vi "TMY_R2_set_angle.vi"() -> ()   [LabVIEW 2023, in "TMY_R2_20250714.lvlib"]
uses:
  TMY_R2_20250714.lvlib
panel:
  out "String":string
  in  "Phi":i32 min=0 max=360
  in  "Theta":i32 min=0 max=360
  in  "COM_No.":string="10"
  out "floder?":bool
  out "standard output":string
  out "standard error":string
  in  "error in":errorcluster
  in  "Func.":enum16{"Theta", "Phi"}(ring)
  out "error out":errorcluster
  # "# 設定角度\ntheta_angle = 10 #大轉盤\nphi_angle = 20 #DUT轉盤"
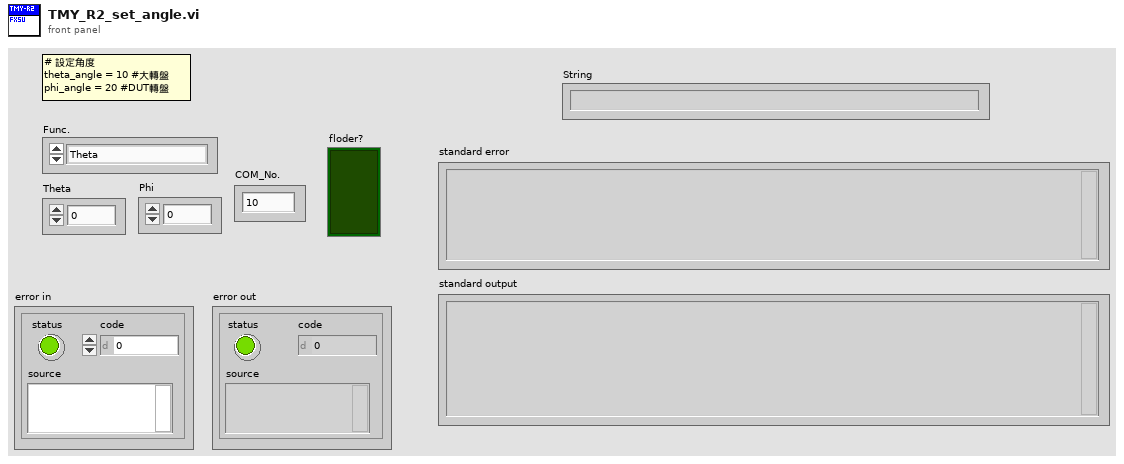
[diagram p1: front panel]
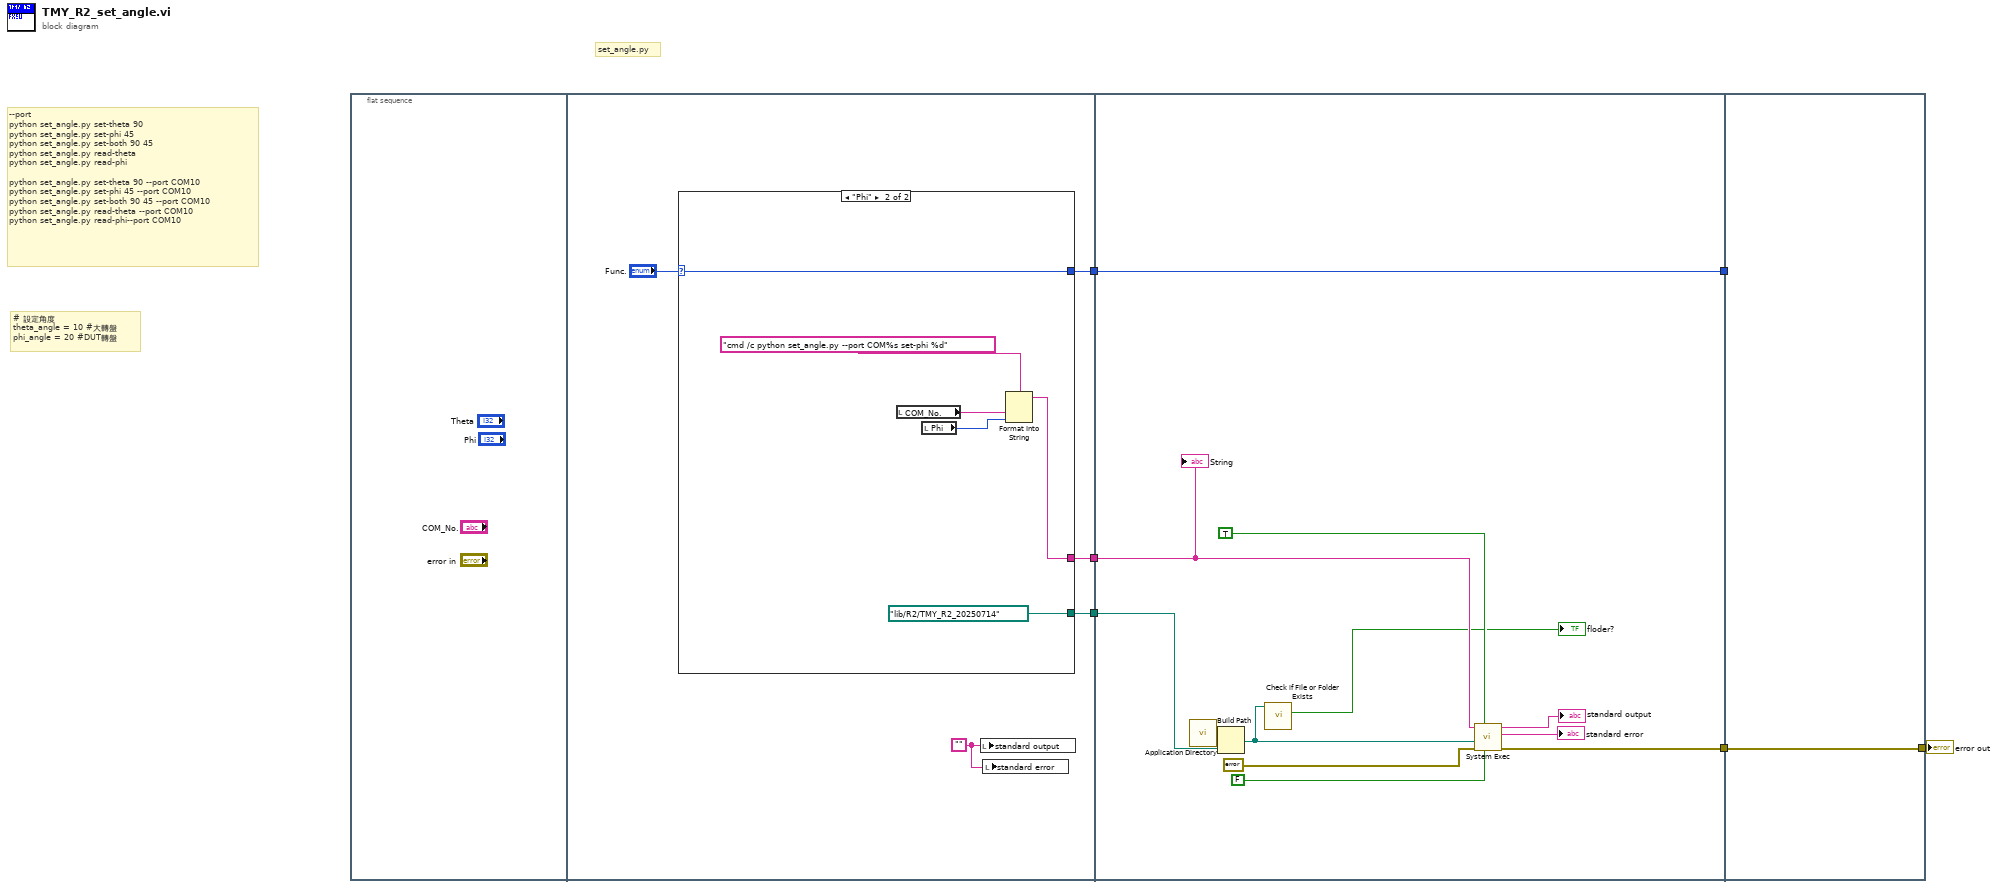
[diagram p0: block diagram]
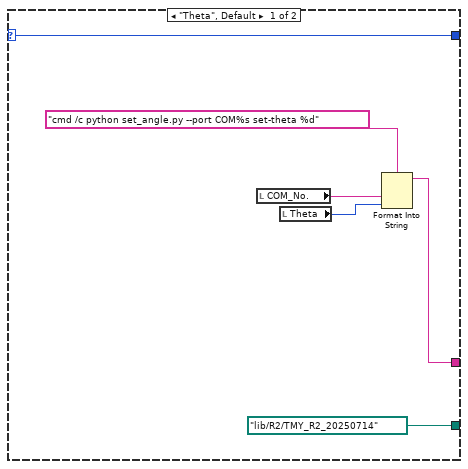
[diagram p2: hidden frame]
diagram:
  # "# 設定角度\ntheta_angle = 10 #大轉盤\nphi_angle = 20 #DUT轉盤"
  # "--port\npython set_angle.py set-theta 90 \npython set_angle.py set-phi 45 \npython set_angle.py set-both 90 45 \npython set_angle.py read-theta \npython set_angle.py read-phi\n\npython set_angle.py set-theta 90 --port COM10\npython set_angle.py set-phi 45 --port COM10\npython set_angle.py set-both 90 45 --port COM10\npython set_angle.py read-theta --port COM10\npython set_angle.py read-phi--port COM10"
  # "set_angle.py"
  n1 = flat-sequence {
    tunnel: [w10] -> w6
    tunnel: [w9] -> w5
    tunnel: [w7] -> w4
    tunnel: [w29] -> w3
    tunnel: w6 -> [w27]
    tunnel: w5 -> [w26]
    tunnel: [w24] -> w2
    tunnel: w4 -> [w24]
    tunnel: [w36] -> w1
    tunnel: w3 -> [w36]
    tunnel: w2 -> [_]
    frame #0 {
    }
    frame #1 {
      w11 = ""
      n2 = case shown="\"Phi\"" "Func." {
        selector: "Func." -> [w16 w22]
        tunnel: [w14 w20] -> w10
        tunnel: [path "lib/R2/TMY_R2_20250714" ("name or relative path") path "lib/R2/TMY_R2_20250714" ("name or relative path")] -> w9
        tunnel: [w16 w22] -> w7
        frame "Theta", Default {
          n3 = local read "COM_No."() -> (w13:string)
          n4 = local read "Theta"() -> (w12:i32)
          n5 = Format Into String(format string="cmd /c python set_angle.py --port COM%s set-theta %d" ("command line"), w13, w12) -> (resulting string=w14:string)  [unwired: 2 in, 1 out]
        }
        frame "Phi" {
          n6 = local read "COM_No."() -> (w19:string)
          n7 = local read "Phi"() -> (w18:i32)
          n8 = Format Into String(format string="cmd /c python set_angle.py --port COM%s set-phi %d" ("command line"), w19, w18) -> (resulting string=w20:string)  [unwired: 2 in, 1 out]
        }
      }
      n9 = local write "standard output"(w11) -> ()
      n10 = local write "standard error"(w11) -> ()
    }
    frame #2 {
      n11 = call <vilib>:"Application Directory.vi"() -> ("Application Directory"=w32:path)
      n12 = Build Path(base path=w32, name or relative path=w26) -> (appended path=w35:path)
      n13 = call <vilib>:"Check if File or Folder Exists.vi"("path"=w35) -> ("file or folder exists?"=→"floder?":bool)  [unwired: 8 in, 2 out]
      n14 = call <vilib>:"System Exec.vi"("run minimized? (F)"=FALSE, "wait until completion? (T)"=TRUE, "error in (no error)"=errorcluster {"status"=FALSE, "code"=0, "source"=""}, "working directory"=w35, "command line"=w27) -> ("error out"=w29:errorcluster, "standard error"=→"standard error":string, "standard output"=→"standard output":string)  [unwired: 3 in, 1 out]
      "String" <- w27
    }
    frame #3 {
    }
  }
  "error out" <- w1
